vi "Clear buffer.vi"(8 "错误输入（无错误）":errorcluster caption="Error In(No Error)", 11 "CAN Device In":T1={"Device Type"=20, "Device Index"=0, "CANInd"=0, "Baud(E_U)"=1835016} {"Baud(E_U)" items=["1000Kbps"=393219, "800Kbps"=393220, "500Kbps"=393223, "250Kbps"=1835016, "125Kbps"=1835025, "100Kbps"=1441827, "50Kbps"=1835052, "20Kbps"=1441971, "10Kbps"=1835232, "5Kbps"=1835457]; "Device Type" items=["PCI5121"=1, "PCI9810"=2, "USBCAN1"=3, "USBCAN2"=4, "PCI9820"=5, "PCI5110"=7, "PC104CAN"=11, "CANETUDP"=12, "PCI9840B"=14, "PC104C2"=15, "PCI9820I"=16, "CANETTCP"=17, "PCIE9221"=24, "PCI5010U"=19, "USBCAN_E_U"=20, "USBCAN_2E_U"=21, "PCI5020U"=22, "PCIE9120I"=27, "PCIE9110I"=28, "PCIE9140I"=29, "USBCAN-4E-U"=31, "USBCAN-8E-U"=34]}) -> (0 "错误输出":errorcluster caption="Error Out", 3 "CAN Device Out":T1={"Device Type"=20, "Device Index"=0, "CANInd"=0, "Baud(E_U)"=1835016} {"Baud(E_U)" items=["1000Kbps"=393219, "800Kbps"=393220, "500Kbps"=393223, "250Kbps"=1835016, "125Kbps"=1835025, "100Kbps"=1441827, "50Kbps"=1835052, "20Kbps"=1441971, "10Kbps"=1835232, "5Kbps"=1835457]; "Device Type" items=["PCI5121"=1, "PCI9810"=2, "USBCAN1"=3, "USBCAN2"=4, "PCI9820"=5, "PCI5110"=7, "PC104CAN"=11, "CANETUDP"=12, "PCI9840B"=14, "PC104C2"=15, "PCI9820I"=16, "CANETTCP"=17, "PCIE9221"=24, "PCI5010U"=19, "USBCAN_E_U"=20, "USBCAN_2E_U"=21, "PCI5020U"=22, "PCIE9120I"=27, "PCIE9110I"=28, "PCIE9140I"=29, "USBCAN-4E-U"=31, "USBCAN-8E-U"=34]})   [LabVIEW 2020, in "ZLGCAN.lvclass"]
uses:
  ZLGCAN.lvclass
  Device.ctl
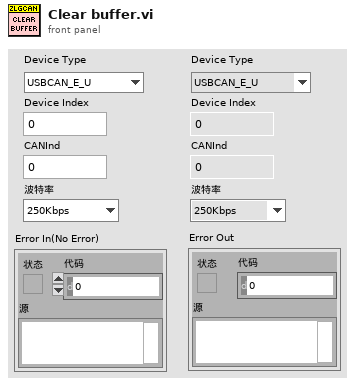
[diagram p1: front panel]
types:
  T1 = typedef "ZLGCAN.lvclass/Device.ctl" = cluster{"Device Type":u32, "Device Index":u32, "CANInd":u32, "Baud(E_U)":u32}
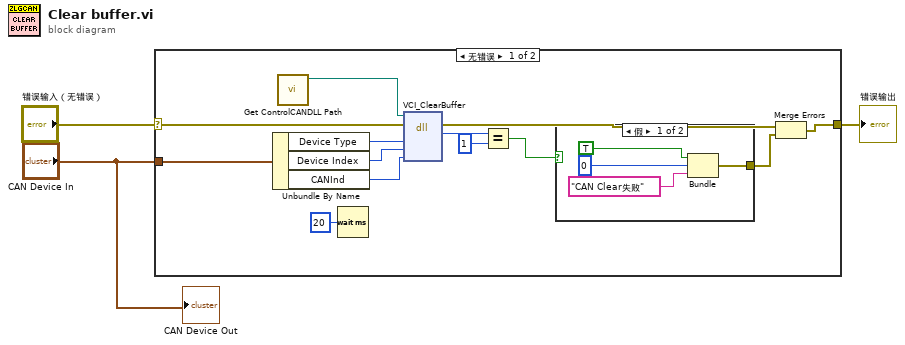
[diagram p0: block diagram]
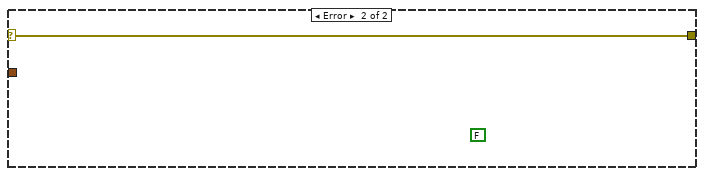
[diagram p3: hidden frame]
diagram:
  n1 = case shown="无错误" "错误输入（无错误）" {
    selector: "错误输入（无错误）" -> [w6 w21]
    tunnel: [w13 w21] -> w2
    tunnel: "CAN Device In" -> [w5 _]
    frame No Error {
      n2 = Unbundle By Name(w5) -> ("Device Type"=w10:u32, "Device Index"=w9:u32, "CANInd"=w8:u32)
      n3 = call "Get ControlCANDLL Path.vi"() -> ("拆分的路径"=w4:path)  [unwired: 10 in, 1 out]
      n4 = Wait (ms)(milliseconds to wait=u32 20 ("等待时间（毫秒）")) -> ()  [unwired: 1 out]
      n5 = dll-call lib="D:/SourceCode/eDMTPlus Monitor/trunk/support/ZLG CAN/ControlCAN.dll" fn="VCI_ClearBuffer"(path in=w4, error in=w6, "DeviceType"=w10, "DeviceInd"=w9, "CANInd"=w8) -> (error out=w12:errorcluster, "返回类型"=w11:u32)  [unwired: 4 in, 1 out]
      n6 = Equal?(x=w11, y=u32 1) -> (x = y?=w14:bool)
      n7 = case shown="假" w14 {
        tunnel: [w17 _] -> w15
        frame False {
          n8 = Bundle("status"=TRUE, "code"=0, "消息"="CAN Clear失败") -> (w17:cluster{"status":bool, "code":i32, "消息":string})  [unwired: 1 in]
        }
        frame True {
        }
      }
      n9 = Merge Errors(w12, w15) -> (w13:errorcluster)
    }
    frame Error {
      (unwired) FALSE
    }
  }
  "错误输出" <- w2
  "CAN Device Out" <- "CAN Device In"
